vi "Write Repository Path.vi"(8 "error in (no error)":errorcluster, 10 "Repository Path":path, 11 "Git in":refnum<class "Git.lvclass">) -> (0 "error out":errorcluster, 3 "Git out":refnum<class "Git.lvclass">)   [LabVIEW 2019, in "Git.lvclass"]
uses:
  Git.lvclass
  Git.lvclass/Git.ctl
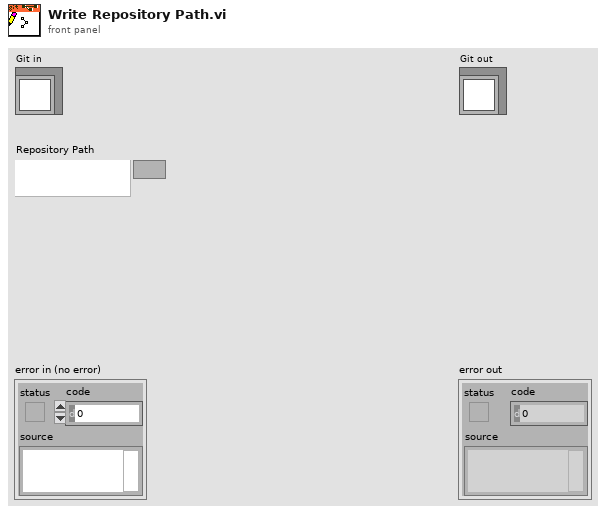
[diagram p1: front panel]
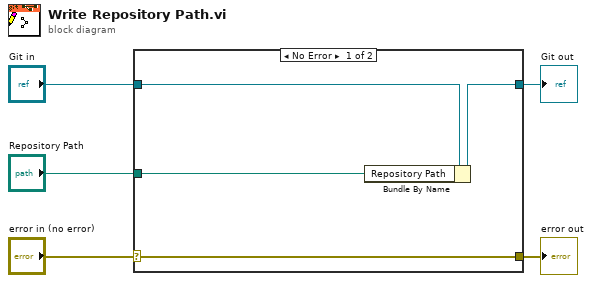
[diagram p0: block diagram]
diagram:
  n1 = case shown="No Error" "error in (no error)" {
    selector: "error in (no error)" -> [w9 w10]
    tunnel: [w9 w10] -> w4
    tunnel: [w7 w11] -> w2
    tunnel: "Git in" -> [w8 w11]
    tunnel: "Repository Path" -> [w6 _]
    frame No Error {
      n2 = Bundle By Name(cluster=w8, "Repository Path"=w6) -> (w7:refnum<class "Git.lvclass">)
    }
    frame Error {
    }
  }
  "error out" <- w4
  "Git out" <- w2
